vi "save_high_score.vi"(11 "Your Score":i32) -> (1 "Top Ten High Score 2":T1(array[cluster])=[{"Placing"=1.0, "Name"="", "Score"=0.0, "Date"=""}, {"Placing"=2.0, "Name"="", "Score"=0.0, "Date"=""}, {"Placing"=3.0, "Name"="", "Score"=0.0, "Date"=""}, {"Placing"=4.0, "Name"="", "Score"=0.0, "Date"=""}, {"Placing"=5.0, "Name"="", "Score"=0.0, "Date"=""}, {"Placing"=6.0, "Name"="", "Score"=0.0, "Date"=""}, {"Placing"=7.0, "Name"="", "Score"=0.0, "Date"=""}, {"Placing"=8.0, "Name"="", "Score"=0.0, "Date"=""}, {"Placing"=9.0, "Name"="", "Score"=0.0, "Date"=""}, {"Placing"=10.0, "Name"="", "Score"=0.0, "Date"=""}])   [LabVIEW 2014]
panel:
  in  "Enter player name: \n(less than 16 characters)":string="Player 1"
  in  "OK Button":bool
  out "new":bool
  out "first time":bool
  out "new index":i32
  out "path":path
  in  "Top Ten High Score":T1(array[cluster])=[{"Placing"=1.0, "Name"="", "Score"=0.0, "Date"=""}, {"Placing"=2.0, "Name"="", "Score"=0.0, "Date"=""}, {"Placing"=3.0, "Name"="", "Score"=0.0, "Date"=""}, {"Placing"=4.0, "Name"="", "Score"=0.0, "Date"=""}, {"Placing"=5.0, "Name"="", "Score"=0.0, "Date"=""}, {"Placing"=6.0, "Name"="", "Score"=0.0, "Date"=""}, {"Placing"=7.0, "Name"="", "Score"=0.0, "Date"=""}, {"Placing"=8.0, "Name"="", "Score"=0.0, "Date"=""}, {"Placing"=9.0, "Name"="", "Score"=0.0, "Date"=""}, {"Placing"=10.0, "Name"="", "Score"=0.0, "Date"=""}]
  out "score":i32[](array[numeric])
  out "entered name":string
  out "String":string
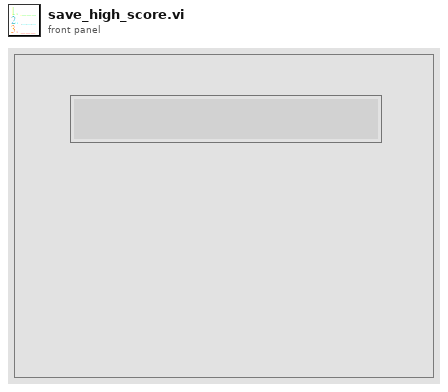
[diagram p1: front panel]
types:
  T1 = cluster{"Placing":dbl, "Name":string, "Score":dbl, "Date":string}[]
  T2 = enum16{"open", "replace", "create", "open or create", "replace or create", "replace or create with confirmation"}
  T3 = enum8{"Enabled", "Disabled", "Disabled and Grayed Out"}
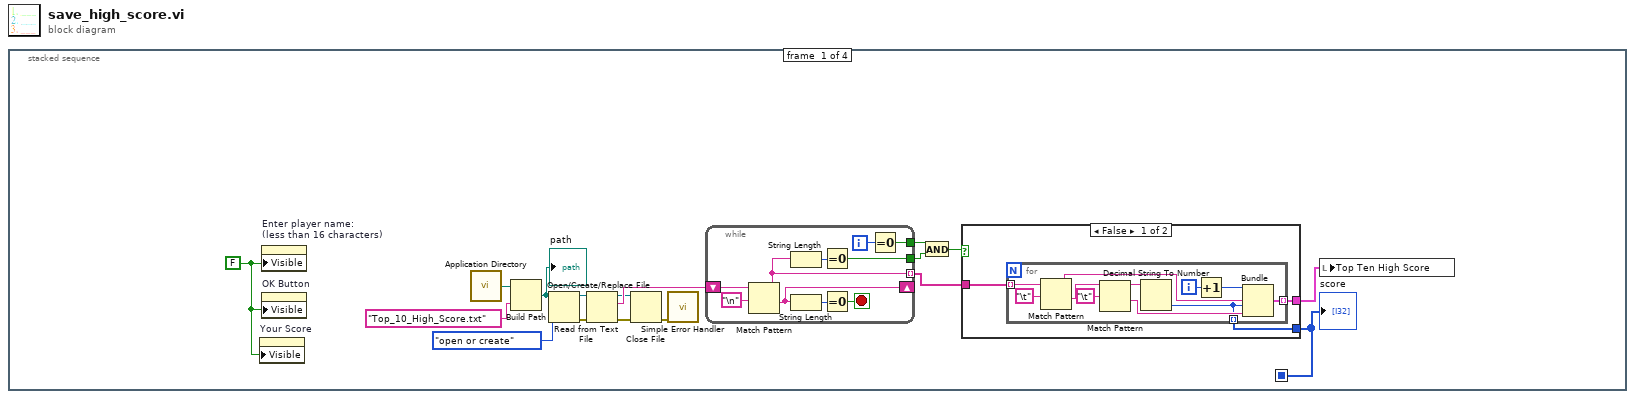
[diagram p0: block diagram]
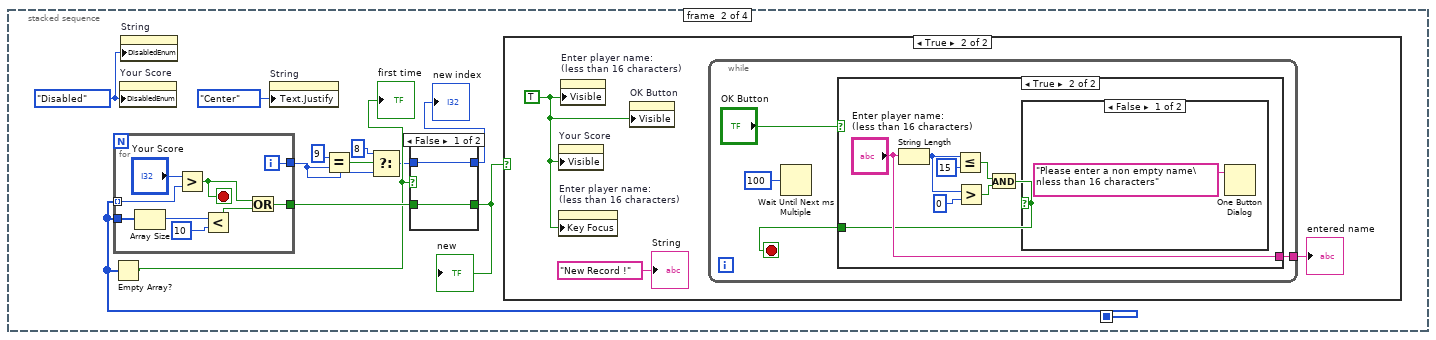
[diagram p3: hidden frame]
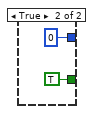
[diagram p4: hidden frame]
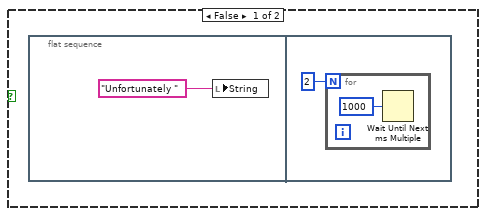
[diagram p5: hidden frame]
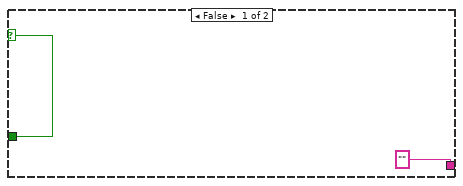
[diagram p6: hidden frame]
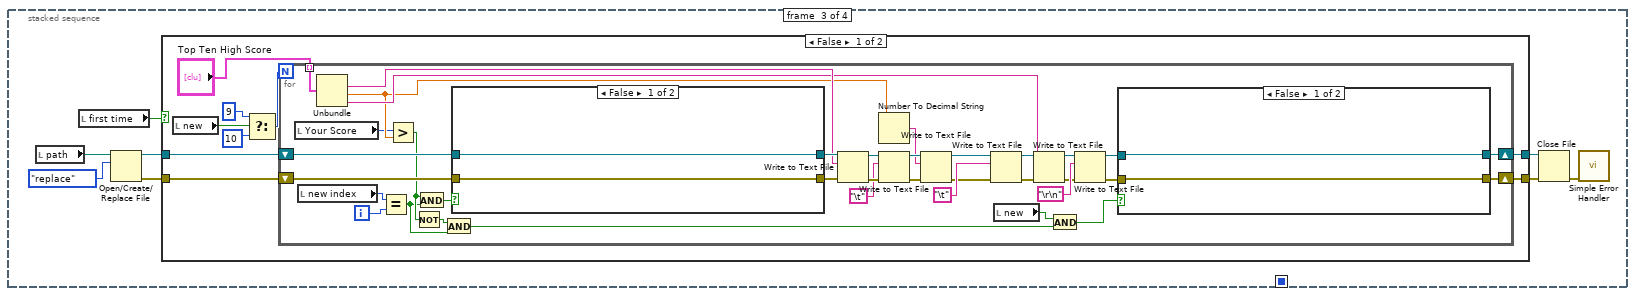
[diagram p8: hidden frame]
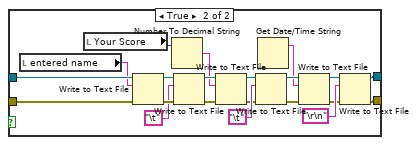
[diagram p9: hidden frame]
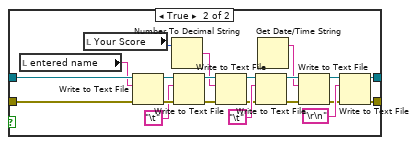
[diagram p10: hidden frame]
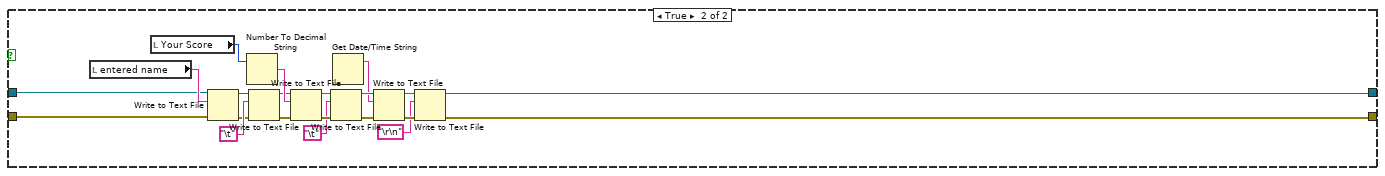
[diagram p11: hidden frame]
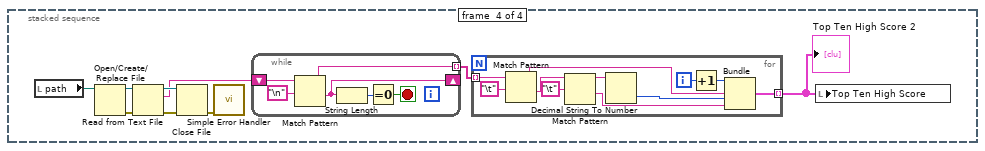
[diagram p12: hidden frame]
diagram:
  n1 = stacked-sequence {
    seq-local: [w7 _ _ _] -> [_ w50 _ _]
    frame #0 {
      w2 = FALSE
      n2 = property on="Your Score" class="DigNum (strict)"("Visible"=w2) -> ()  [unwired: 2 in, 2 out]
      n3 = property on="Enter player name: \n(less than 16 characters)" class="Str"("Visible"=w2) -> ()  [unwired: 2 in, 2 out]
      n4 = property on="OK Button" class="Bool"("Visible"=w2) -> ()  [unwired: 2 in, 2 out]
      n5 = call <vilib>:"Application Directory.vi"() -> ("Application Directory"=w1:path)
      n6 = Build Path(base path=w1, name or relative path="Top_10_High_Score.txt") -> (appended path=w15:path)
      "path" <- w15
      n7 = Open/Create/Replace File(file path (use dialog)=w15, operation (0:open)=T2."open or create") -> (refnum out=w8:refnum<file>, error out=w9:errorcluster)  [unwired: 4 in, 1 out]
      n8 = Read from Text File(file (use dialog)=w8, error in=w9) -> (refnum out=w11:refnum<file>, text=w13:string, error out=w10:errorcluster)  [unwired: 2 in, 1 out]
      n9 = Close File(refnum=w11, error in=w10) -> (error out=w12:errorcluster)  [unwired: 1 out]
      n10 = call <vilib>:"Simple Error Handler.vi"("error in (no error)"=w12) -> ()  [unwired: 4 in, 5 out]
      n11 = while {
        shift-right: [w37] -> _
        shift-left: w13 -> [w41]
        tunnel: [w35] -> w16 mode=indexing
        tunnel: [w34] -> w5
        tunnel: [w32] -> w4
        i -> [w33]
        stop <- w39 stop-if-true
        n12 = Match Pattern(string=w41, regular expression="\n") -> (before substring=w35:string, after substring=w37:string)  [unwired: 1 in, 2 out]
        n13 = String Length(string=w35) -> (length=w36:i32)
        n14 = String Length(string=w37) -> (length=w40:i32)
        n15 = Equal To 0?(x=w36) -> (x = 0?=w34:bool)
        n16 = Equal To 0?(x=w40) -> (x = 0?=w39:bool)
        n17 = Equal To 0?(x=w33) -> (x = 0?=w32:bool)
      }
      n18 = And(x=w4, y=w5) -> (x .and. y?=w3:bool)
      n19 = case shown="False" w3 {
        tunnel: [w20 _] -> w17
        tunnel: w16 -> [w19 _]
        tunnel: [w18 _] -> w7
        frame False {
          n20 = for {
            tunnel: w19 -> [w31] mode=indexing
            tunnel: [w28] -> w20 mode=indexing
            tunnel: [w21] -> w18 mode=indexing
            i -> [w27]
            n21 = Match Pattern(string=w31, regular expression="\t") -> (before substring=w29:string, after substring=w25:string)  [unwired: 1 in, 2 out]
            n22 = Match Pattern(string=w25, regular expression="\t") -> (before substring=w23:string, after substring=w22:string)  [unwired: 1 in, 2 out]
            n23 = Decimal String To Number(string=w23) -> (number=w21:i32)  [unwired: 2 in, 1 out]
            n24 = Increment(x=w27) -> (x+1=w26:i32)
            n25 = Bundle(w26, w29, w21, w22) -> (w28:cluster{i32, string, i32, string})  [unwired: 1 in]
          }
        }
        frame True {
        }
      }
      "score" <- w7
      n26 = local write "Top Ten High Score"(w17) -> ()
    }
    frame #1 {
      w42 = T3."Disabled" ("Disabled")
      n27 = Empty Array?(array=w50) -> (empty?=w49:bool)
      "first time" <- w49
      n28 = for {
        tunnel: w50 -> [w85] mode=indexing
        tunnel: w50 -> [w84]
        tunnel: [w80] -> w53
        tunnel: [w79] -> w45
        i -> [w79]
        stop <- w81 stop-if-true
        n29 = Array Size(array=w84) -> (size(s)=w78:i32)
        n30 = Greater?(x="Your Score", y=w85) -> (0:w81:bool)
        n31 = Less?(x=w78, y=10 ("x")) -> (x < y?=w83:bool)
        n32 = Or(x=w81, y=w83) -> (x .or. y?=w80:bool)
      }
      n33 = property on="Your Score" class="DigNum (strict)"("DisabledEnum"=w42) -> ()  [unwired: 2 in, 2 out]
      n34 = property on="String" class="Str"("DisabledEnum"=w42) -> ()  [unwired: 2 in, 2 out]
      n35 = property on="String" class="Str"("Text.Justify"=enum16{"Left", "Center", "Right"}."Center" ("Text.Justification")) -> ()  [unwired: 2 in, 2 out]
      n36 = Equal?(x=9, y=w45) -> (x = y?=w47:bool)
      n37 = Select(t=8, s=w47, f=w45) -> (s? t:f=w44:i32)
      n38 = case shown="False" w49 {
        tunnel: w53 -> [w54 _]
        tunnel: w44 -> [w55 _]
        tunnel: [w55 0] -> w52
        tunnel: [w54 TRUE] -> w51
        frame False {
        }
        frame True {
        }
      }
      "new index" <- w52
      "new" <- w51
      n39 = case shown="True" w51 {
        frame False {
          n40 = flat-sequence {
            frame #0 {
              n41 = local write "String"("Unfortunately " ("String")) -> ()
            }
            frame #1 {
              n42 = for {
                N: 2 -> [_]
                n43 = Wait Until Next ms Multiple(millisecond multiple=u32 1000) -> ()  [unwired: 1 out]
              }
            }
          }
        }
        frame True {
          w61 = TRUE
          n44 = property on="Your Score" class="DigNum (strict)"("Visible"=w61) -> ()  [unwired: 2 in, 2 out]
          n45 = property on="Enter player name: \n(less than 16 characters)" class="Str"("Key Focus"=w61) -> ()  [unwired: 2 in, 2 out]
          n46 = property on="Enter player name: \n(less than 16 characters)" class="Str"("Visible"=w61) -> ()  [unwired: 2 in, 2 out]
          n47 = property on="OK Button" class="Bool"("Visible"=w61) -> ()  [unwired: 2 in, 2 out]
          n48 = while {
            tunnel: [w65] -> w63
            stop <- w66 stop-if-true
            n49 = Wait Until Next ms Multiple(millisecond multiple=u32 100) -> ()  [unwired: 1 out]
            n50 = case shown="True" "OK Button" {
              selector: "OK Button" -> [w69 _]
              tunnel: [w69 w70] -> w66
              tunnel: ["" ("enter player name:") "Enter player name: \n(less than 16 characters)"] -> w65
              frame False {
              }
              frame True {
                n51 = String Length(string="Enter player name: \n(less than 16 characters)") -> (length=w74:i32)
                n52 = Less Or Equal?(x=w74, y=15) -> (x <= y?=w72:bool)
                n53 = Greater?(x=w74, y=0) -> (0:w71:bool)
                n54 = And(x=w72, y=w71) -> (x .and. y?=w70:bool)
                n55 = case shown="False" w70 {
                  frame False {
                    n56 = One Button Dialog(message="Please enter a non empty name\nless than 16 characters") -> ()  [unwired: 1 in, 1 out]
                  }
                  frame True {
                  }
                }
              }
            }
          }
          "entered name" <- w63
          "String" <- "New Record !" ("String")
        }
      }
    }
    frame #2 {
      n57 = local read "path"() -> (w88:path)
      n58 = local read "first time"() -> (w87:bool)
      n59 = Open/Create/Replace File(file path (use dialog)=w88, operation (0:open)=T2."replace") -> (refnum out=w94:refnum<file>, error out=w93:errorcluster)  [unwired: 4 in, 1 out]
      n60 = case shown="False" w87 {
        tunnel: w94 -> [w103 w190]
        tunnel: w93 -> [w102 w189]
        tunnel: [w101 w188] -> w91
        tunnel: [w100 w187] -> w90
        frame False {
          n61 = local read "new"() -> (w98:bool)
          n62 = Select(t=9, s=w98, f=10) -> (s? t:f=w97:i32)
          n63 = for {
            N: w97 -> [_]
            shift-right: [w108] -> w101
            shift-left: w103 -> [w137]
            shift-right: [w107] -> w100
            shift-left: w102 -> [w136]
            tunnel: "Top Ten High Score" -> [w135] mode=indexing
            i -> [w139]
            n64 = local read "Your Score"() -> (w114:i32)
            n65 = local read "new index"() -> (w138:i32)
            n66 = Unbundle(w135) -> ("Name"=w118:string, "Score"=w115:dbl, "Date"=w117:string)  [unwired: 1 out]
            n67 = Equal?(x=w138, y=w139) -> (x = y?=w111:bool)
            n68 = Greater?(x=w114, y=w115) -> (0:w113:bool)
            n69 = Not(x=w113) -> (.not. x?=w112:bool)
            n70 = And(x=w113, y=w111) -> (x .and. y?=w116:bool)
            n71 = And(x=w112, y=w111) -> (x .and. y?=w105:bool)
            n72 = case shown="False" w116 {
              tunnel: w137 -> [w163 w185]
              tunnel: w136 -> [w164 w184]
              tunnel: [w163 w183] -> w120
              tunnel: [w164 w182] -> w119
              frame False {
              }
              frame True {
                n73 = local read "entered name"() -> (w165:string)
                n74 = local read "Your Score"() -> (w166:i32)
                n75 = Write to Text File(file (use dialog)=w185, text=w165, error in=w184) -> (refnum out=w181:refnum<file>, error out=w180:errorcluster)  [unwired: 1 in, 1 out]
                n76 = Number To Decimal String(number=w166) -> (decimal integer string=w176:string)  [unwired: 1 in]
                n77 = Write to Text File(file (use dialog)=w181, text="\t", error in=w180) -> (refnum out=w178:refnum<file>, error out=w177:errorcluster)  [unwired: 1 in, 1 out]
                n78 = Write to Text File(file (use dialog)=w178, text=w176, error in=w177) -> (refnum out=w173:refnum<file>, error out=w172:errorcluster)  [unwired: 1 in, 1 out]
                n79 = Write to Text File(file (use dialog)=w173, text="\t", error in=w172) -> (refnum out=w171:refnum<file>, error out=w170:errorcluster)  [unwired: 1 in, 1 out]
                n80 = Get Date/Time String() -> (date string=w167:string)  [unwired: 3 in, 1 out]
                n81 = Write to Text File(file (use dialog)=w171, text=w167, error in=w170) -> (refnum out=w169:refnum<file>, error out=w168:errorcluster)  [unwired: 1 in, 1 out]
                n82 = Write to Text File(file (use dialog)=w169, text="\r\n", error in=w168) -> (refnum out=w183:refnum<file>, error out=w182:errorcluster)  [unwired: 1 in, 1 out]
              }
            }
            n83 = Write to Text File(file (use dialog)=w120, text=w118, error in=w119) -> (refnum out=w134:refnum<file>, error out=w133:errorcluster)  [unwired: 1 in, 1 out]
            n84 = Number To Decimal String(number=w115) -> (decimal integer string=w121:string)  [unwired: 1 in]
            n85 = Write to Text File(file (use dialog)=w134, text="\t", error in=w133) -> (refnum out=w131:refnum<file>, error out=w130:errorcluster)  [unwired: 1 in, 1 out]
            n86 = Write to Text File(file (use dialog)=w131, text=w121, error in=w130) -> (refnum out=w127:refnum<file>, error out=w126:errorcluster)  [unwired: 1 in, 1 out]
            n87 = Write to Text File(file (use dialog)=w127, text="\t", error in=w126) -> (refnum out=w125:refnum<file>, error out=w124:errorcluster)  [unwired: 1 in, 1 out]
            n88 = local read "new"() -> (w106:bool)
            n89 = Write to Text File(file (use dialog)=w125, text=w117, error in=w124) -> (refnum out=w123:refnum<file>, error out=w122:errorcluster)  [unwired: 1 in, 1 out]
            n90 = And(x=w106, y=w105) -> (x .and. y?=w104:bool)
            n91 = Write to Text File(file (use dialog)=w123, text="\r\n", error in=w122) -> (refnum out=w110:refnum<file>, error out=w109:errorcluster)  [unwired: 1 in, 1 out]
            n92 = case shown="False" w104 {
              tunnel: w110 -> [w140 w162]
              tunnel: w109 -> [w141 w161]
              tunnel: [w140 w160] -> w108
              tunnel: [w141 w159] -> w107
              frame False {
              }
              frame True {
                n93 = local read "entered name"() -> (w142:string)
                n94 = local read "Your Score"() -> (w143:i32)
                n95 = Write to Text File(file (use dialog)=w162, text=w142, error in=w161) -> (refnum out=w158:refnum<file>, error out=w157:errorcluster)  [unwired: 1 in, 1 out]
                n96 = Number To Decimal String(number=w143) -> (decimal integer string=w153:string)  [unwired: 1 in]
                n97 = Write to Text File(file (use dialog)=w158, text="\t", error in=w157) -> (refnum out=w155:refnum<file>, error out=w154:errorcluster)  [unwired: 1 in, 1 out]
                n98 = Write to Text File(file (use dialog)=w155, text=w153, error in=w154) -> (refnum out=w150:refnum<file>, error out=w149:errorcluster)  [unwired: 1 in, 1 out]
                n99 = Write to Text File(file (use dialog)=w150, text="\t", error in=w149) -> (refnum out=w148:refnum<file>, error out=w147:errorcluster)  [unwired: 1 in, 1 out]
                n100 = Get Date/Time String() -> (date string=w144:string)  [unwired: 3 in, 1 out]
                n101 = Write to Text File(file (use dialog)=w148, text=w144, error in=w147) -> (refnum out=w146:refnum<file>, error out=w145:errorcluster)  [unwired: 1 in, 1 out]
                n102 = Write to Text File(file (use dialog)=w146, text="\r\n", error in=w145) -> (refnum out=w160:refnum<file>, error out=w159:errorcluster)  [unwired: 1 in, 1 out]
              }
            }
          }
        }
        frame True {
          n103 = local read "entered name"() -> (w192:string)
          n104 = local read "Your Score"() -> (w191:i32)
          n105 = Write to Text File(file (use dialog)=w190, text=w192, error in=w189) -> (refnum out=w193:refnum<file>, error out=w194:errorcluster)  [unwired: 1 in, 1 out]
          n106 = Number To Decimal String(number=w191) -> (decimal integer string=w198:string)  [unwired: 1 in]
          n107 = Write to Text File(file (use dialog)=w193, text="\t", error in=w194) -> (refnum out=w196:refnum<file>, error out=w197:errorcluster)  [unwired: 1 in, 1 out]
          n108 = Write to Text File(file (use dialog)=w196, text=w198, error in=w197) -> (refnum out=w201:refnum<file>, error out=w202:errorcluster)  [unwired: 1 in, 1 out]
          n109 = Write to Text File(file (use dialog)=w201, text="\t", error in=w202) -> (refnum out=w203:refnum<file>, error out=w204:errorcluster)  [unwired: 1 in, 1 out]
          n110 = Get Date/Time String() -> (date string=w186:string)  [unwired: 3 in, 1 out]
          n111 = Write to Text File(file (use dialog)=w203, text=w186, error in=w204) -> (refnum out=w205:refnum<file>, error out=w206:errorcluster)  [unwired: 1 in, 1 out]
          n112 = Write to Text File(file (use dialog)=w205, text="\r\n", error in=w206) -> (refnum out=w188:refnum<file>, error out=w187:errorcluster)  [unwired: 1 in, 1 out]
        }
      }
      n113 = Close File(refnum=w91, error in=w90) -> (error out=w89:errorcluster)  [unwired: 1 out]
      n114 = call <vilib>:"Simple Error Handler.vi"("error in (no error)"=w89) -> ()  [unwired: 4 in, 5 out]
    }
    frame #3 {
      n115 = local read "path"() -> (w208:path)
      n116 = Open/Create/Replace File(file path (use dialog)=w208) -> (refnum out=w215:refnum<file>, error out=w214:errorcluster)  [unwired: 5 in, 1 out]
      n117 = Read from Text File(file (use dialog)=w215, error in=w214) -> (refnum out=w212:refnum<file>, text=w210:string, error out=w213:errorcluster)  [unwired: 2 in, 1 out]
      n118 = Close File(refnum=w212, error in=w213) -> (error out=w211:errorcluster)  [unwired: 1 out]
      n119 = call <vilib>:"Simple Error Handler.vi"("error in (no error)"=w211) -> ()  [unwired: 4 in, 5 out]
      n120 = while {
        shift-right: [w227] -> _
        shift-left: w210 -> [w232]
        tunnel: [w231] -> w209 mode=indexing
        stop <- w229 stop-if-true
        n121 = Match Pattern(string=w232, regular expression="\n") -> (before substring=w231:string, after substring=w227:string)  [unwired: 1 in, 2 out]
        n122 = String Length(string=w227) -> (length=w230:i32)
        n123 = Equal To 0?(x=w230) -> (x = 0?=w229:bool)
      }
      n124 = for {
        tunnel: w209 -> [w226] mode=indexing
        tunnel: [w222] -> w207 mode=indexing
        i -> [w221]
        n125 = Match Pattern(string=w226, regular expression="\t") -> (before substring=w223:string, after substring=w219:string)  [unwired: 1 in, 2 out]
        n126 = Match Pattern(string=w219, regular expression="\t") -> (before substring=w217:string, after substring=w216:string)  [unwired: 1 in, 2 out]
        n127 = Decimal String To Number(string=w217) -> (number=w224:i32)  [unwired: 2 in, 1 out]
        n128 = Increment(x=w221) -> (x+1=w220:i32)
        n129 = Bundle(w220, w223, w224, w216) -> (w222:cluster{i32, string, i32, string})  [unwired: 1 in]
      }
      "Top Ten High Score 2" <- w207
      n130 = local write "Top Ten High Score"(w207) -> ()
    }
  }
